vi "steerer set.vi"(0 "Injector image X  -":dbl format="%#_4g", 1 "Injector image X +":dbl format="%#_4g", 2 "Injector image Y  -":dbl format="%#_4g", 3 "Injector image Y +":dbl format="%#_4g") -> (8 "Steerer X":dbl format="%#_4g", 9 "Steerer Y":dbl format="%#_4g")   [LabVIEW 2016, in "Low energy.lvlib"]
doc: "this vi takes the positive and negative signals from a steerer and displays the set value for a steerer"
uses:
  Low energy.lvlib
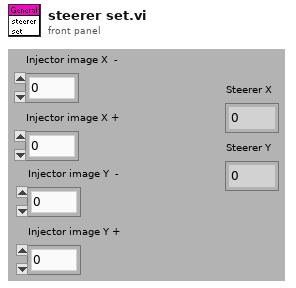
[diagram p1: front panel]
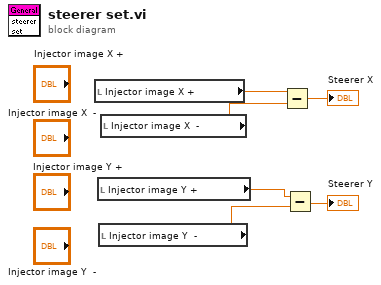
[diagram p0: block diagram]
diagram:
  n1 = local read "Injector image X +"() -> (w1:dbl)
  n2 = local read "Injector image Y +"() -> (w3:dbl)
  n3 = local read "Injector image Y  -"() -> (w4:dbl)
  n4 = local read "Injector image X  -"() -> (w2:dbl)
  n5 = Subtract(x=w1, y=w2) -> (x-y=→"Steerer X":dbl)
  n6 = Subtract(x=w3, y=w4) -> (x-y=→"Steerer Y":dbl)
